vi "error_window.vi"(0 "Source":string, 1 "Start":i32[](array[numeric]), 2 "Length":i32[](array[numeric]), 3 "code":i32, 4 "Show Link":bool, 5 "Details":string="reason for problem", 6 "calling_vi":refnum<vi>, 7 "dialog type":T2, 9 "Error or Warning":bool, 11 "contname":string="Continue", 12 "stopname":string="Stop", 13 "okname":string="OK", 14 "Tag Found?":T1) -> (15 "stop event propagated":bool)   [LabVIEW 2015, in "lv-dialog-interfaces.lvlib"]
uses:
  lv-dialog-interfaces.lvlib
  <vilib>/Utility/error.llb/DialogTypeEnum.ctl
  <vilib>/Utility/error.llb/TagReturnType.ctl
  _controls/hmi_references.ctl
  lv-dialog/api/v1/public/_controls/configuration.ctl
  _controls/dialog_type.ctl
  <vilib>/event_ctls.llb/eventvkey.ctl
  lv-dialog/api/v1/v1.lvlib
panel:
  in  "Search ni.com":bool
  in  "truncated message":string="(source truncated)"
  in  "truncated & CH message":string="(source truncated; see Context Help window)"
  out "Source of Error":string
  out "scrollbar text":string
  in  "Test for size":string
  out "text":string
  out "?":bool=TRUE
  in  "continue":bool
  in  "stop":bool
  in  "continue":bool
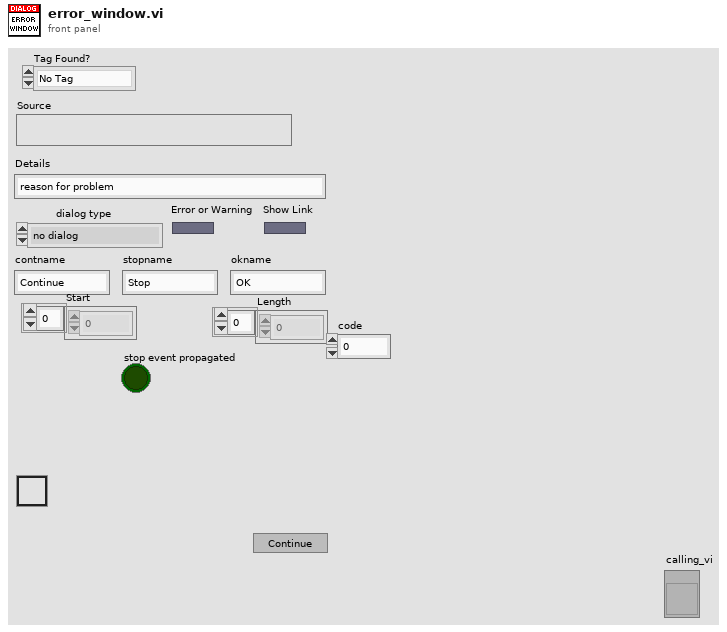
[diagram p1: front panel]
types:
  T1 = typedef "TagReturnType.ctl" = enum16{"No Tag", "<err>", "<append>"}
  T2 = typedef "DialogTypeEnum.ctl" = enum16{"no dialog", "OK message", "continue or stop message", "auto error handling dialog", "OK message + warnings", "continue/stop + warnings"}
  T3 = typedef "lv-dialog-interfaces.lvlib/dialog_type.ctl" = enum16{"null", "one_button", "two_button", "three_button", "confirmation", "busy_wait", "error", "busy_wait_embed", "combo_box", "data_entry_string", "data_entry_numeric"}
  T4 = typedef "lv-dialog.lvlib/v1.lvlib/configuration.ctl" = cluster{"dialog_text":string, "boolean_text_1":string, "boolean_text_2":string, "boolean_text_3":string, "inner_color":u32, "outer_color":u32, "wait_s":dbl, "error_status":bool, "error_source":string, "error_details":string, "string []":string[], "custom_entry":bool}
  T5 = typedef "lv-dialog-interfaces.lvlib/hmi_references.ctl" = cluster{"vi_reference":refnum<vi>, "caller":refnum<vi>, "dialog":refnum<vi>, "button_1":refnum<vi>, "button_2":refnum<vi>, "button_3":refnum<vi>, "busy":refnum<vi>, "error_glyph":refnum<vi>, "error_source":refnum<vi>, "error_text":refnum<vi>, "combo_box":refnum<vi>}
  T6 = typedef "eventvkey.ctl" = enum16{"ASCII", "Enter", "Return", "Shift", "Ctrl", "Alt", "Cmd", "Opt", "Caps", "NumLock", "Clear", "Break", "Up", "Down", "Left", "Right", "Insert", "Delete", "Home", "End", "PageUp", "PageDown", "Escape", "Help", "Pause", "ScrollLock", "F1", "F2", "F3", "F4", "F5", "F6", "F7", "F8", "F9", "F10", "F11", "F12", "F13", "F14", "F15", "F16", "F17", "F18", "F19", "F20", "F21", "F22", "F23", "F24", "Play", "VolumeUp", "VolumeDown", "Mute", "Two Byte Char"}
  T7 = typedef "LVRectTypeDef.ctl" = cluster{"Left":i16, "Top":i16, "Right":i16, "Bottom":i16}
  T8 = cluster{"Control":bool, "Shift":bool, "Key":string}
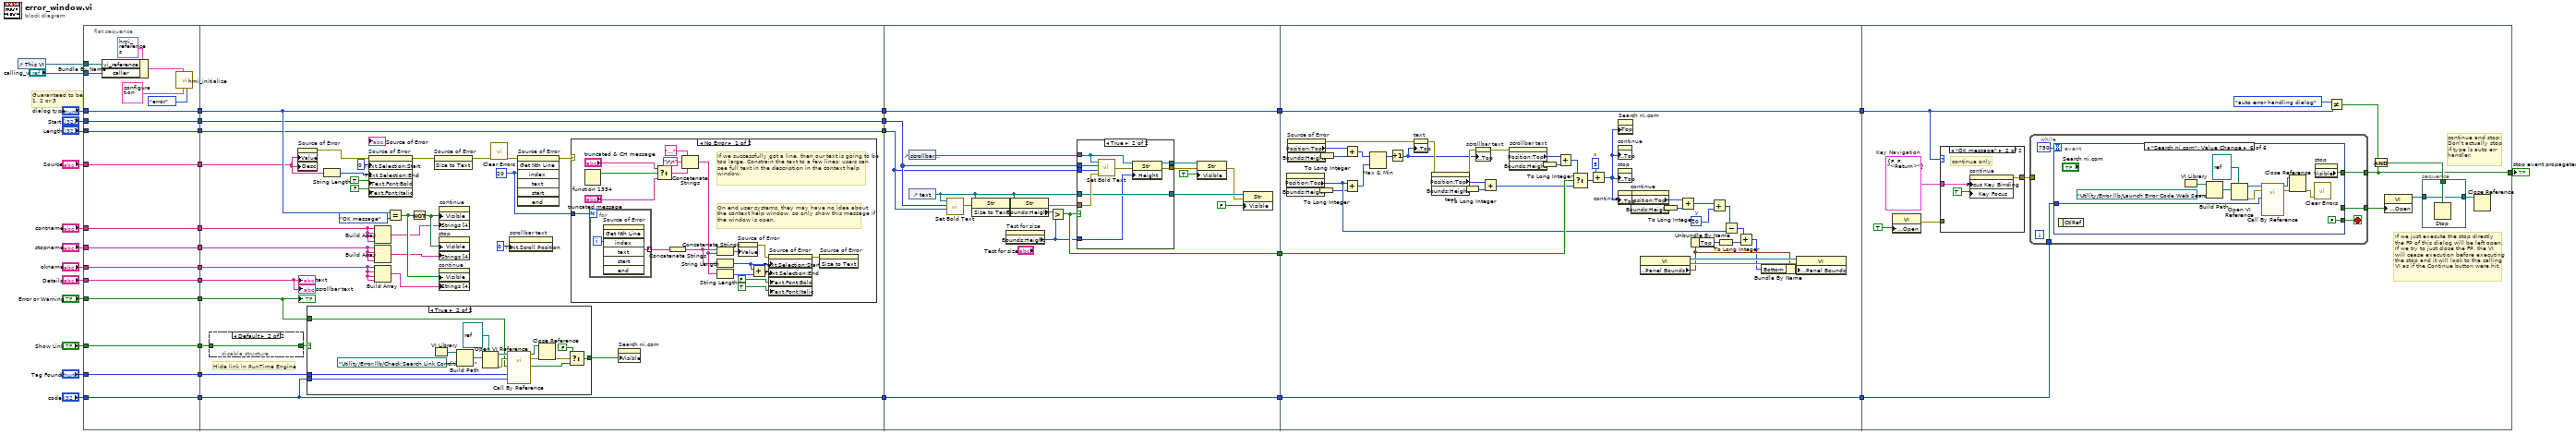
[diagram p0: block diagram]
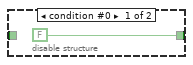
[diagram p2: hidden frame]
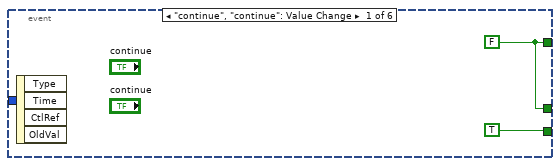
[diagram p6: hidden frame]
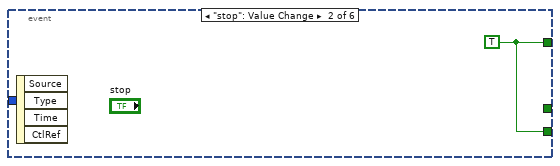
[diagram p7: hidden frame]
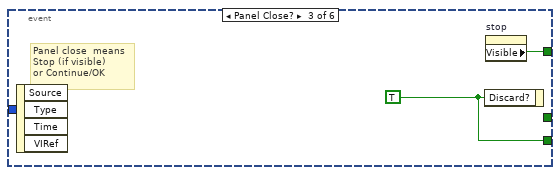
[diagram p8: hidden frame]
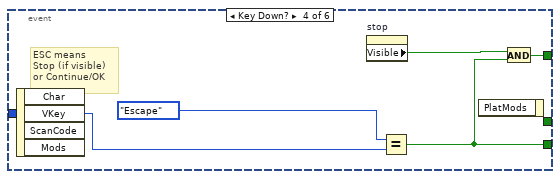
[diagram p9: hidden frame]
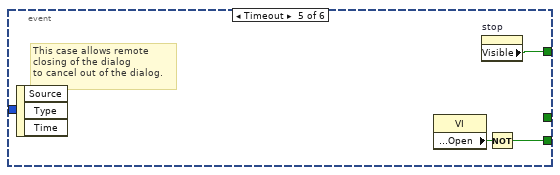
[diagram p10: hidden frame]
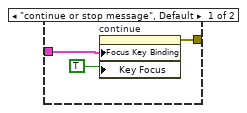
[diagram p11: hidden frame]
diagram:
  # "Guaranteed to be\n1, 2 or 3"
  n1 = control-ref of="This VI"() -> (w14:refnum<vi>)
  n2 = flat-sequence {
    tunnel: "calling_vi" -> [w38]
    tunnel: w14 -> [w39]
    tunnel: "Tag Found?" -> [w43]
    tunnel: "code" -> [w44]
    tunnel: "Show Link" -> [w45]
    tunnel: "Length" -> [w46]
    tunnel: "Start" -> [w47]
    tunnel: "Error or Warning" -> [w48]
    tunnel: "Details" -> [w49]
    tunnel: "Source" -> [w50]
    tunnel: "okname" -> [w51]
    tunnel: "stopname" -> [w52]
    tunnel: "contname" -> [w53]
    tunnel: "dialog type" -> [w54]
    tunnel: [w54] -> w12
    tunnel: [w53] -> w11
    tunnel: [w52] -> w10
    tunnel: [w51] -> w9
    tunnel: [w50] -> w8
    tunnel: [w49] -> w7
    tunnel: [w48] -> w6
    tunnel: [w47] -> w5
    tunnel: [w46] -> w4
    tunnel: [w45] -> w3
    tunnel: [w44] -> w2
    tunnel: [w43] -> w1
    tunnel: [w68] -> w35
    tunnel: [w63] -> w24
    tunnel: [w62] -> w23
    tunnel: [w57] -> w16
    tunnel: w12 -> [w68]
    tunnel: w11 -> [w67]
    tunnel: w10 -> [w66]
    tunnel: w9 -> [w65]
    tunnel: w8 -> [w61]
    tunnel: w7 -> [w64]
    tunnel: w6 -> [w55]
    tunnel: w5 -> [w63]
    tunnel: w4 -> [w62]
    tunnel: w3 -> [w60]
    tunnel: w2 -> [w57]
    tunnel: w1 -> [w58]
    tunnel: w35 -> [w126]
    tunnel: [w126] -> w34
    tunnel: [w132] -> w33
    tunnel: w24 -> [w125]
    tunnel: w23 -> [w124]
    tunnel: [w123] -> w17
    tunnel: w16 -> [w123]
    tunnel: w34 -> [w161]
    tunnel: [w161] -> w32
    tunnel: w33 -> [w195]
    tunnel: [w154] -> w18
    tunnel: w17 -> [w154]
    tunnel: [w197] -> w36
    tunnel: w32 -> [w199]
    tunnel: w18 -> [w196]
    frame #0 {
      n3 = Bundle By Name(cluster=T5 {"vi_reference"=refnum, "caller"=refnum, "dialog"=refnum, "button_1"=refnum, "button_2"=refnum, "button_3"=refnum, "busy"=refnum, "error_glyph"=refnum, "error_source"=refnum, "error_text"=refnum, "combo_box"=refnum} ("references"), "vi_reference"=w39, "caller"=w38) -> (w37:T5)
      n4 = call "hmi_initialize.vi"("dialog_type"=dialog_type."error", "configuration"=T4 {"dialog_text"="", "boolean_text_1"="", "boolean_text_2"="", "boolean_text_3"="", "inner_color"=16711680, "outer_color"=6618880, "wait_s"=nan, "error_status"=FALSE, "error_source"="", "error_details"="", "string []"=[], "custom_entry"=FALSE}, "references"=w37) -> ()  [unwired: 8 in, 1 out]
    }
    frame #1 {
      w75 = u32 20 ("index")
      # "Hide link in RunTime Engine"
      n5 = disable-structure shown="Default" {
        disable-tunnel: w60 -> [_ w87]
        disable-tunnel: [FALSE ("Show Link") w87] -> w59
        frame condition #0 {
        }
        frame condition #1 (active) {
        }
      }
      n6 = property on="Source of Error" class="Str"("Value"=w61, "Desc"=w61) -> (error out=w74:errorcluster)  [unwired: 2 in, 1 out]
      n7 = case shown="True" w59 {
        tunnel: [_ w95] -> w56
        tunnel: w58 -> [_ w94]
        tunnel: w57 -> [_ w93]
        tunnel: w55 -> [_ w92]
        frame False {
        }
        frame True {
          n8 = VI Library() -> (path=w101:path)
          n9 = Build Path(base path=w101, name or relative path=path "Utility/Error.llb/Check Search Link Conditions.vi") -> (appended path=w102:path)
          n10 = Open VI Reference(type specifier VI Refnum (for type only)=refnum<vi> refnum, vi path=w102) -> (vi reference=w98:refnum<vi>, error out=w100:errorcluster)  [unwired: 4 in]
          n11 = call-by-ref "?"(reference=w98, error in=w100, "Error Code"=w93, "Tag Found?"=w94, "Error or Warning?"=w92) -> (reference out=w91:refnum<vi>, error out=w90:errorcluster, "Display Link?"=w97:bool)  [unwired: 8 in]
          n12 = Close Reference(reference=w91, error in (no error)=w90) -> (error out=w89:errorcluster)
          n13 = Select(t=FALSE, s=w89, f=w97) -> (s? t:f=w95:bool)
        }
      }
      n14 = String Length(string=w61) -> (length=w71:i32)
      n15 = property on="Source of Error" class="Str"(error in=w74, "Text.Selection:Start"=u32 0, "Text.Selection:End"=w71, "Text.Font:Bold"=TRUE, "Text.Font:Italic"=FALSE) -> (error out=w73:errorcluster)  [unwired: 1 in, 1 out]
      n16 = Build Array(w67, w67, w67, w67) -> (w83:string[])
      n17 = Build Array(w66, w66, w66, w66) -> (w82:string[])
      n18 = Build Array(w65, w65, w65, w65) -> (w81:string[])
      n19 = Equal?(x=w68, y=DialogTypeEnum."OK message" ("dialog type")) -> (x = y?=w85:bool)
      n20 = Not(x=w85) -> (.not. x?=w84:bool)
      n21 = invoke on="Source of Error" class="Str" method="Size to Text"(error in=w73) -> (error out=w78:errorcluster)  [unwired: 2 in, 2 out]
      n22 = property on="continue" class="Bool"("Visible"=w84, "Strings [4]"=w83) -> ()  [unwired: 2 in, 2 out]
      n23 = property on="stop" class="Bool"("Visible"=w84, "Strings [4]"=w82) -> ()  [unwired: 2 in, 2 out]
      n24 = property on="continue" class="Bool"("Visible"=w85, "Strings [4]"=w81) -> ()  [unwired: 2 in, 2 out]
      n25 = call <vilib>:"Clear Errors.vi"("error in (no error)"=w78) -> ("error out"=w77:errorcluster)  [unwired: 5 in, 1 out]
      n26 = property on="scrollbar text" class="Str"("Text.Scroll Position"=u32 0) -> ()  [unwired: 2 in, 2 out]
      n27 = invoke on="Source of Error" class="Str" method="Get Nth Line"(error in=w77, "index"=w75) -> (error out=w76:errorcluster)  [unwired: 5 in, 6 out]
      n28 = case shown="No Error" w76 {
        tunnel: w75 -> [w120 _]
        frame No Error {
          # "If we successfully got a line, then our text is going to be too large. Constrain the text to a few lines; users can see full text in the description in the context help window."
          # "On end user systems, they may have no idea about\nthe context help window, so only show this message if\nthe window is open."
          n29 = fn#1354() -> (1:w110:bool)  [unwired: 1 out]
          n30 = for {
            N: w120 -> [_]
            tunnel: [w121] -> w118 mode=indexing
            i -> [w122]
            n31 = invoke on="Source of Error" class="Str" method="Get Nth Line"("index"=w122) -> ("text"=w121:string)  [unwired: 6 in, 6 out]
          }
          n32 = Select(t="truncated & CH message", s=w110, f="truncated message") -> (s? t:f=w107:string)
          n33 = Concatenate Strings(w118) -> (w117:string)
          n34 = Concatenate Strings("..." ("string"), "\r\n", w107) -> (w104:string)
          n35 = Concatenate Strings(w117, w104) -> (w119:string)
          n36 = String Length(string=w117) -> (length=w112:i32)
          n37 = String Length(string=w104) -> (length=w109:i32)
          n38 = property on="Source of Error" class="Str"("Value"=w119) -> (error out=w114:errorcluster)  [unwired: 2 in, 1 out]
          n39 = Add(x=w112, y=w109) -> (x+y=w111:i32)
          n40 = property on="Source of Error" class="Str"(error in=w114, "Text.Selection:Start"=w112, "Text.Selection:End"=w111, "Text.Font:Bold"=FALSE, "Text.Font:Italic"=TRUE) -> (error out=w113:errorcluster)  [unwired: 1 in, 1 out]
          n41 = invoke on="Source of Error" class="Str" method="Size to Text"(error in=w113) -> ()  [unwired: 2 in, 3 out]
        }
        frame Error {
          # "An error at this point means that there is no line to fetch. That's good. We do not want the text getting too large."
        }
      }
      n42 = property on="Search ni.com" class="Bool"("Visible"=w56) -> ()  [unwired: 2 in, 2 out]
      "?" <- w55
      "scrollbar text" <- w64
      "text" <- w64
    }
    frame #2 {
      n43 = control-ref of="scrollbar text"() -> (w135:refnum<vi>)
      n44 = control-ref of="text"() -> (w127:refnum<vi>)
      n45 = call <vilib>:"Set Bold Text.vi"("Length"=w124, "Start"=w125, "text"=w127) -> ("error out"=w130:errorcluster)  [unwired: 3 in]
      n46 = invoke class="Str" method="Size to Text"(reference=w127, error in=w130) -> (error out=w131:errorcluster)  [unwired: 1 in, 2 out]
      n47 = property on="Test for size" class="Str"() -> ("Bounds:Height"=w129:u32)  [unwired: 2 in, 2 out]
      n48 = property class="Str"(reference=w127, error in=w131) -> (error out=w139:errorcluster, "Bounds:Height"=w140:u32)  [unwired: 1 out]
      n49 = Greater?(x=w140, y=w129) -> (0:w132:bool)
      n50 = case shown="True" w132 {
        tunnel: w139 -> [w143 w152]
        tunnel: w125 -> [_ w151]
        tunnel: w124 -> [_ w150]
        tunnel: [w143 w147] -> w128
        tunnel: w127 -> [w142 w149]
        tunnel: [w142 w144] -> w137
        tunnel: [w141 w149] -> w136
        tunnel: w135 -> [w141 w145]
        tunnel: w129 -> [_ w148]
        frame False {
        }
        frame True {
          n51 = call <vilib>:"Set Bold Text.vi"("error in"=w152, "Length"=w150, "Start"=w151, "text"=w145) -> ("error out"=w146:errorcluster)  [unwired: 2 in]
          n52 = property class="Str"(reference=w145, error in=w146, "Height"=w148) -> (reference out=w144:refnum<vi>, error out=w147:errorcluster)
        }
      }
      n53 = property class="Str"(reference=w137, error in=w128, "Visible"=TRUE ("Defer Panel Updates")) -> (error out=w133:errorcluster)  [unwired: 1 out]
      n54 = property class="Str"(reference=w136, error in=w133, "Visible"=FALSE ("Defer Panel Updates")) -> ()  [unwired: 2 out]
    }
    frame #3 {
      w182 = 20  # y
      w187 = 5  # x
      n55 = property class="Bool"() -> ("Position:Top"=w177:i32, "Bounds:Height"=w192:u32)  [unwired: 2 in, 2 out]
      n56 = property on="Source of Error" class="Str"() -> (error out=w162:errorcluster, "Position:Top"=w164:i32, "Bounds:Height"=w163:u32)  [unwired: 2 in, 1 out]
      n57 = To Long Integer(number=w192) -> (32bit integer=w160:i32)
      n58 = To Long Integer(number=w163) -> (32bit integer=w159:i32)
      n59 = Add(x=w164, y=w159) -> (x+y=w194:i32)
      n60 = Add(x=w177, y=w160) -> (x+y=w193:i32)
      n61 = Max & Min(x=w194, y=w193) -> (max(x,y)=w191:i32)  [unwired: 1 out]
      n62 = Increment(x=w191) -> (x+1=w170:i32)
      n63 = property on="text" class="Str"(error in=w162, "Position:Top"=w170) -> (error out=w172:errorcluster)  [unwired: 1 in, 1 out]
      n64 = property on="text" class="Str"(error in=w172) -> (error out=w171:errorcluster, "Position:Top"=w169:i32, "Bounds:Height"=w168:u32)  [unwired: 1 in, 1 out]
      n65 = To Long Integer(number=w168) -> (32bit integer=w158:i32)
      n66 = property on="scrollbar text" class="Str"(error in=w171, "Position:Top"=w170) -> (error out=w190:errorcluster)  [unwired: 1 in, 1 out]
      n67 = Add(x=w169, y=w158) -> (x+y=w166:i32)
      n68 = property on="scrollbar text" class="Str"(error in=w190) -> ("Position:Top"=w189:i32, "Bounds:Height"=w188:u32)  [unwired: 1 in, 2 out]
      n69 = To Long Integer(number=w188) -> (32bit integer=w157:i32)
      n70 = Add(x=w189, y=w157) -> (x+y=w167:i32)
      n71 = Select(t=w167, s=w195, f=w166) -> (s? t:f=w165:i32)
      n72 = Add(x=w187, y=w165) -> (x+y=w153:i32)
      n73 = property on="continue" class="Bool"("Position:Top"=w153) -> ()  [unwired: 2 in, 2 out]
      n74 = property on="stop" class="Bool"("Position:Top"=w153) -> ()  [unwired: 2 in, 2 out]
      n75 = property on="continue" class="Bool"("Position:Top"=w153) -> (error out=w186:errorcluster)  [unwired: 2 in, 1 out]
      n76 = property on="Search ni.com" class="Bool"("Top"=w153) -> ()  [unwired: 2 in, 2 out]
      n77 = property on="continue" class="Bool"(error in=w186) -> ("Position:Top"=w184:i32, "Bounds:Height"=w185:u32)  [unwired: 1 in, 2 out]
      n78 = property class="VI"() -> (reference out=w179:refnum<vi>, error out=w180:errorcluster, "Front Panel Window:Panel Bounds"=w176:T7)  [unwired: 2 in]
      n79 = To Long Integer(number=w185) -> (32bit integer=w156:i32)
      n80 = Add(x=w184, y=w156) -> (x+y=w183:i32)
      n81 = Unbundle By Name(w176) -> ("Top"=w174:i16)
      n82 = Add(x=w183, y=w182) -> (x+y=w178:i32)
      n83 = To Long Integer(number=w174) -> (32bit integer=w155:i32)
      n84 = Subtract(x=w178, y=w177) -> (x-y=w175:i32)
      n85 = Add(x=w175, y=w155) -> (x+y=w173:i32)
      n86 = Bundle By Name(cluster=w176, "Bottom"=w173) -> (w181:T7)
      n87 = property class="VI"(reference=w179, error in=w180, "Front Panel Window:Panel Bounds"=w181) -> ()  [unwired: 2 out]
    }
    frame #4 {
      w208 = T8 {"Control"=FALSE, "Shift"=FALSE, "Key"="<Return>"}  # Key Navigation
      # "If we just execute the stop directly\nthe FP of this dialog will be left open.\nIf we try to just close the FP, the VI\nwill cease execution before executing\nthe stop and it will look to the calling\nVI as if the Continue button were hit."
      # "continue and stop;\nDon't actually stop\nif type is auto err\nhandler."
      n88 = property class="VI"("Front Panel Window:Open"=TRUE) -> (error out=w207:errorcluster)  [unwired: 2 in, 1 out]
      n89 = case shown="\"OK message\"" w199 {
        tunnel: w208 -> [w243 w246]
        tunnel: w207 -> [_ _]
        tunnel: [w241 w244] -> w205
        frame "continue or stop message", Default {
          n90 = property on="continue" class="Bool"("Focus Key Binding"=w243, "Key Focus"=TRUE) -> (error out=w241:errorcluster)  [unwired: 2 in, 1 out]
        }
        frame "OK message" {
          # "continue only"
          n91 = property on="continue" class="Bool"("Focus Key Binding"=w246, "Key Focus"=TRUE) -> (error out=w244:errorcluster)  [unwired: 2 in, 1 out]
        }
      }
      n92 = while {
        tunnel: w205 -> [_]
        tunnel: [w214] -> w197
        tunnel: [w213] -> w198
        tunnel: w196 -> [w211]
        stop <- w215 stop-if-true
        n93 = event shown="[5] \"Search ni.com\": Value Change" {
          selector: _ -> [_ _ _ _ _ _]
          dyn-events: _ -> [_ _ _ _ _ _]
          timeout: 750 -> [_ _ _ _ _ _]
          tunnel: [TRUE ("Stop") w218 w220 w221 w226 FALSE ("Discard?")] -> w215
          tunnel: [w217 w218 w219 w224 w228 w240] -> w214
          tunnel: [w217 _ _ _ _ _] -> w213
          tunnel: w211 -> [_ _ _ _ _ w233]
          event "continue", "continue": Value Change {
            w217 = FALSE ("Stop")
            n94 = event-data() -> ()  [unwired: 1 in, 4 out]
          }
          event "stop": Value Change {
            w218 = TRUE
            n95 = event-data() -> ()  [unwired: 1 in, 4 out]
          }
          event Panel Close? {
            w220 = TRUE ("Discard?")
            # "Panel close  means\nStop (if visible)\nor Continue/OK"
            n96 = event-data() -> ()  [unwired: 1 in, 4 out]
            n97 = event-data("Discard?"=w220) -> ()  [unwired: 1 in, 1 out]
            n98 = property on="stop" class="Bool"() -> ("Visible"=w219:bool)  [unwired: 2 in, 2 out]
          }
          event Key Down? {
            # "ESC means\nStop (if visible)\nor Continue/OK"
            n99 = event-data() -> ("VKey"=w223:T6)  [unwired: 1 in, 3 out]
            n100 = property on="stop" class="Bool"() -> ("Visible"=w225:bool)  [unwired: 2 in, 2 out]
            n101 = Equal?(x=eventvkey."Escape", y=w223) -> (x = y?=w221:bool)
            n102 = event-data() -> ()  [unwired: 2 in, 1 out]
            n103 = And(x=w225, y=w221) -> (x .and. y?=w224:bool)
          }
          event Timeout {
            # "This case allows remote\nclosing of the dialog\nto cancel out of the dialog."
            n104 = event-data() -> ()  [unwired: 1 in, 3 out]
            n105 = property class="VI"() -> ("Front Panel Window:Open"=w227:bool)  [unwired: 2 in, 2 out]
            n106 = property on="stop" class="Bool"() -> ("Visible"=w228:bool)  [unwired: 2 in, 2 out]
            n107 = Not(x=w227) -> (.not. x?=w226:bool)
          }
          event "Search ni.com": Value Change {
            n108 = event-data() -> ()  [unwired: 1 in, 1 out]
            n109 = VI Library() -> (path=w235:path)
            n110 = Build Path(base path=w235, name or relative path=path "Utility/Error.llb/Launch Error Code Web Search.vi") -> (appended path=w234:path)
            n111 = Open VI Reference(type specifier VI Refnum (for type only)=refnum<vi> refnum, vi path=w234) -> (vi reference=w238:refnum<vi>, error out=w236:errorcluster)  [unwired: 4 in]
            n112 = call-by-ref "?"(reference=w238, error in=w236, "Code"=w233) -> (reference out=w232:refnum<vi>, error out=w231:errorcluster)  [unwired: 11 in]
            n113 = Close Reference(reference=w232, error in (no error)=w231) -> (error out=w230:errorcluster)
            n114 = call <vilib>:"Clear Errors.vi"("error in (no error)"=w230) -> ()  [unwired: 5 in, 2 out]
            n115 = property on="stop" class="Bool"() -> ("Visible"=w240:bool)  [unwired: 2 in, 2 out]
          }
        }
      }
      n116 = Not Equal?(x=DialogTypeEnum."auto error handling dialog" ("dialog type"), y=w199) -> (x != y?=w204:bool)
      n117 = And(x=w204, y=w197) -> (x .and. y?=w203:bool)
      n118 = property class="VI"("Front Panel Window:Open"=w198) -> (reference out=w201:refnum<vi>)  [unwired: 2 in, 1 out]
      n119 = stacked-sequence {
        tunnel: w201 -> [w209]
        tunnel: w203 -> [w210]
        tunnel: [w209] -> w202
        frame #0 {
          n120 = Stop(stop? (T)=w210) -> ()
        }
      }
      n121 = Close Reference(reference=w202) -> ()  [unwired: 1 in, 1 out]
    }
  }
  "stop event propagated" <- w36
